vi "stdgetdbdataresults1.vi"(6 "connection reference":T1, 7 "type":string="s", 8 "ss ratio":u16(ring) items=["other", "36Cl"], 9 "wheelname":string, 10 "runletter":string, 11 "charge state":i32=2) -> (3 "seq std":dbl[][](array[numeric]), 4 "connection reference out":T1)   [LabVIEW 2016]
uses:
  <vilib>/addons/database/Connection.llb/Conn ObjectReference.ctl
  <vilib>/Analysis/baseanly.llb/Mean (DBL).vi
  <vilib>/addons/database/Connection.llb/Conn Execute.vi
  <vilib>/addons/database/Recordset.llb/Rec Fetch Recordset Data (R).vi
  <vilib>/addons/database/Recordset.llb/Rec Destroy - Connection.vi
  <vilib>/addons/database/NI_Database_API.lvlib
  <vilib>/Analysis/NI_AALBase.lvlib
panel:
  out "concatenated string":string
  out "seq result 2":dbl
  out "sorted array":dbl[](array[numeric])
  out "Array":dbl[][](array[numeric])
  out "position std result":string[][](array[string])
  out "std data":dbl[][][](array[numeric])
  out "seq result":dbl
  in  "SQL query 2":string
  out "error out 2":errorcluster
  out "sample data":string[][](array[string])
  out "recordset data":variant[][](array[variant])
  out "error out":errorcluster
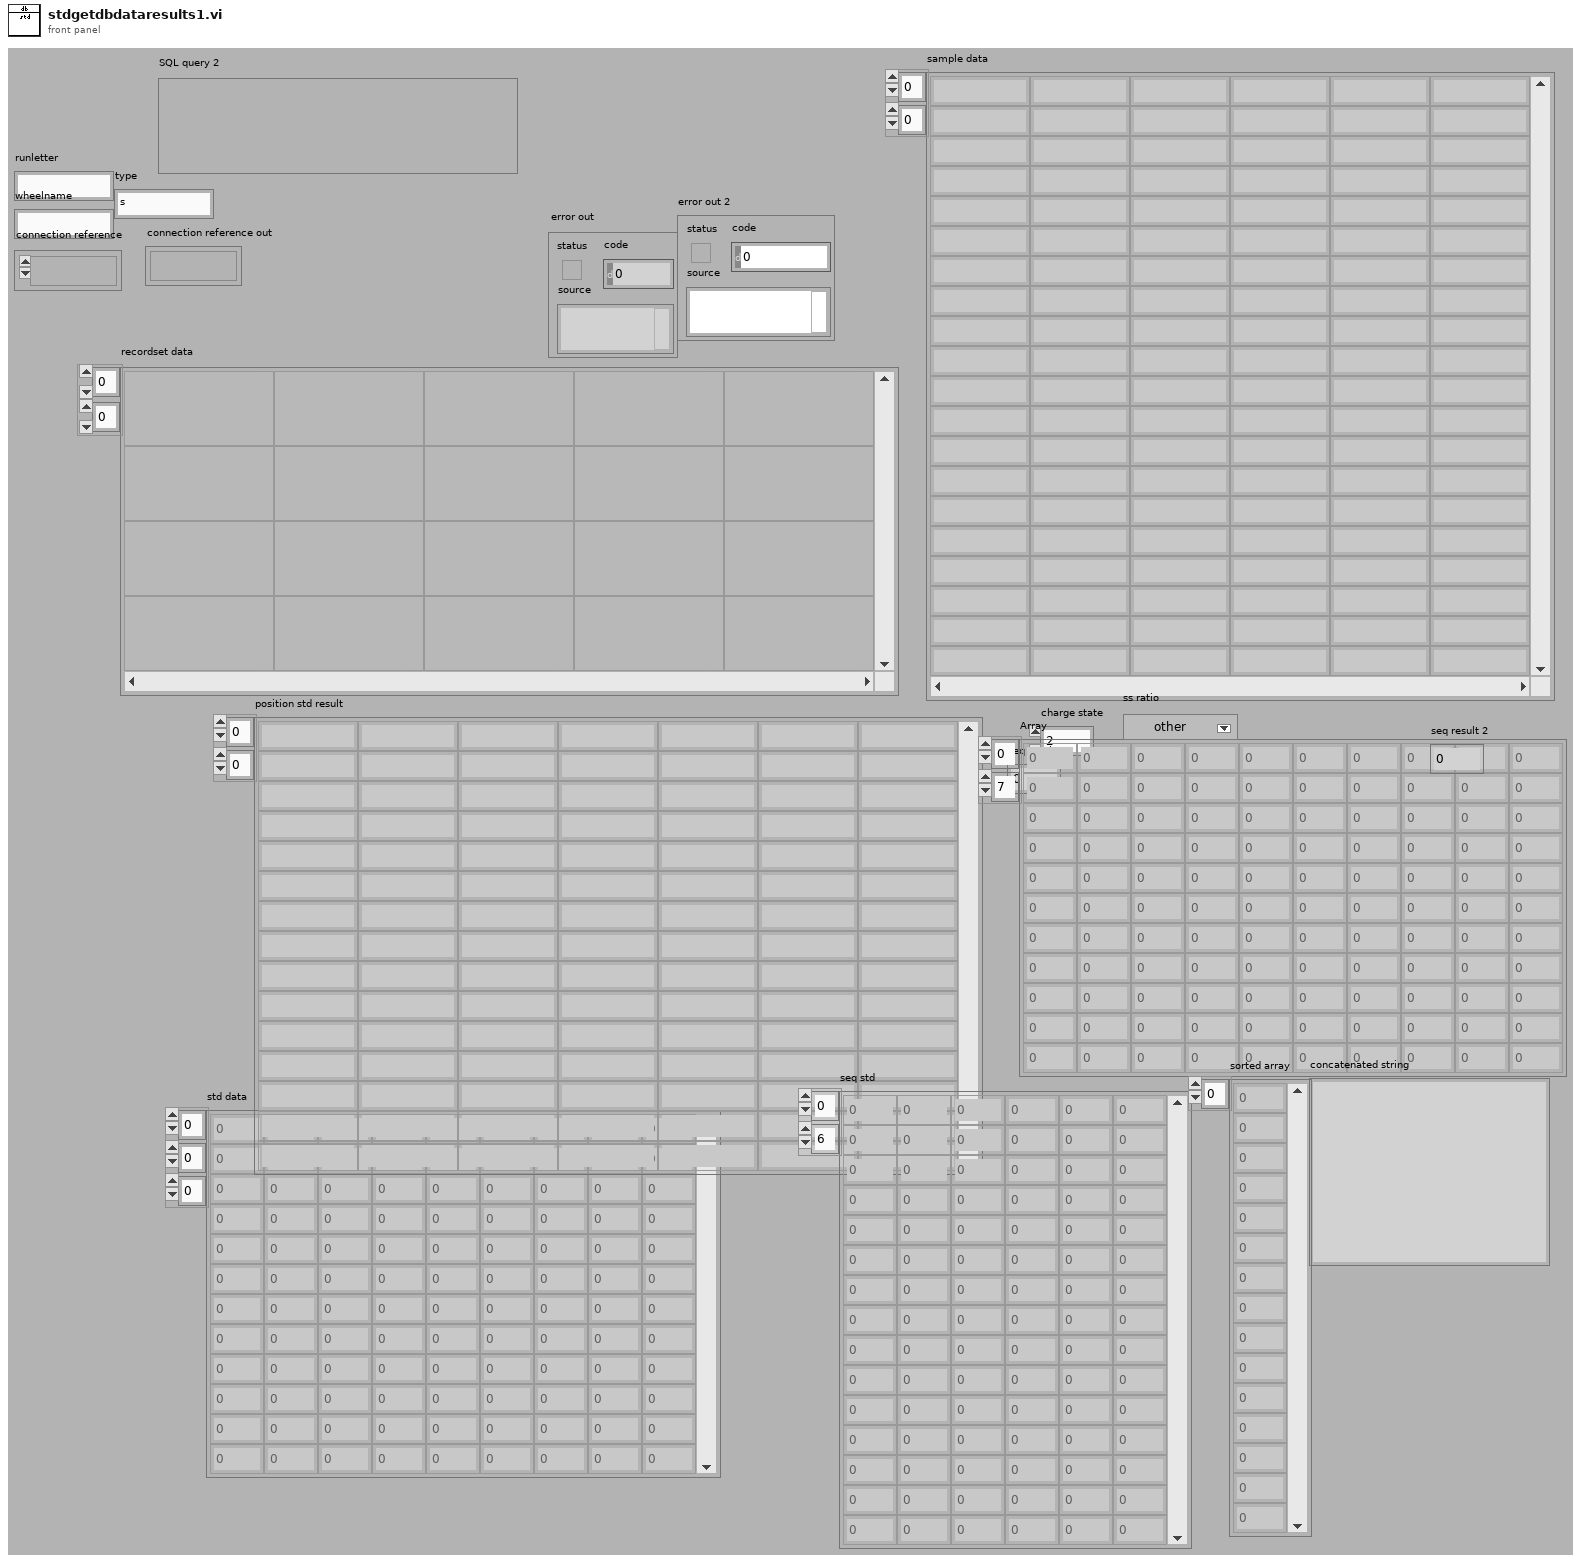
[diagram p1: front panel]
types:
  T1 = typedef "NI_Database_API.lvlib/Conn ObjectReference.ctl" = refnum<k1>
  T2 = typedef "NI_Database_API.lvlib/Rec ObjectReference.ctl" = refnum<k1>
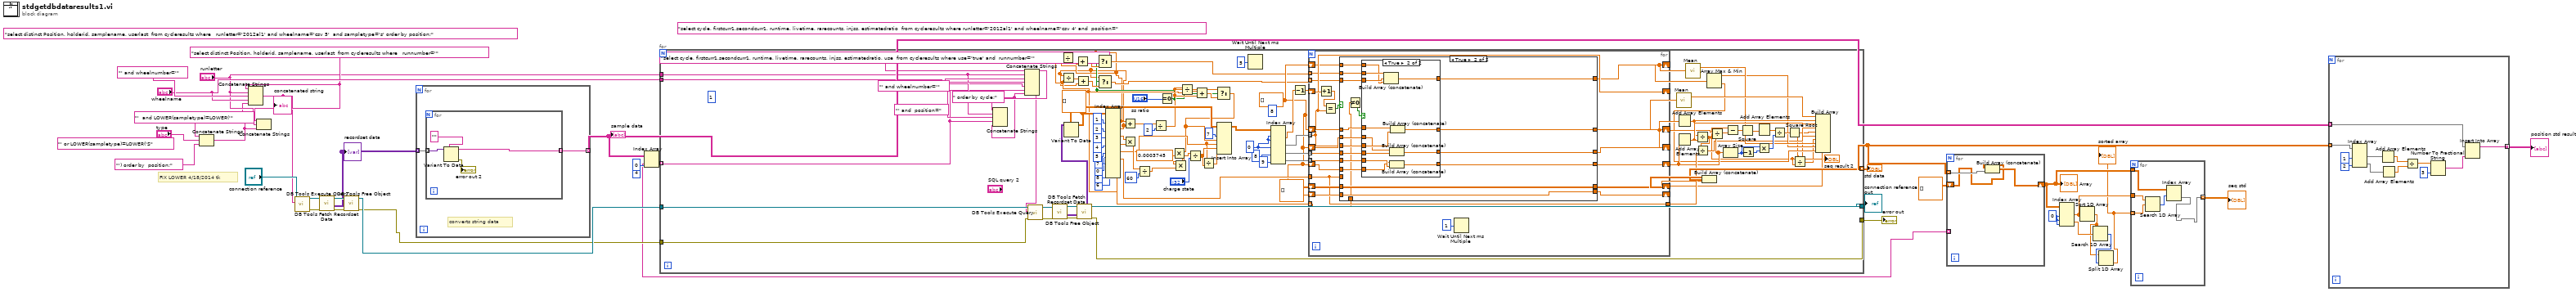
[diagram p0: block diagram]
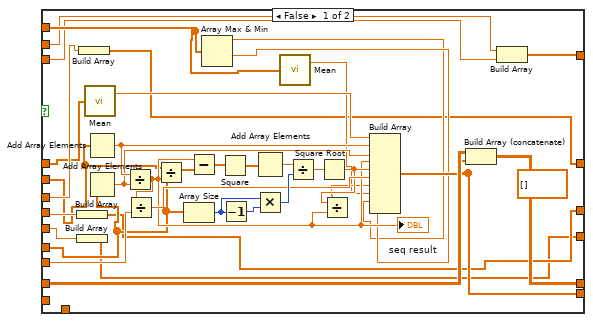
[diagram p2: hidden frame]
diagram:
  (unwired) "' or LOWER(sampletype)=LOWER('S" ("string")
  (unwired) "select cycle, firstcurr1,secondcurr1, runtime, livetime, rarecounts, injss, estimatedratio  from cycleresults where runletter='2012al1' and wheelname='csv 4' and  position=" ("SQL query 3")
  (unwired) "select distinct Position, holderid, samplename, userlast  from cycleresults where   runletter='2012al1' and wheelname='csv 5'  and sampletype='s' order by position;" ("SQL query get data name")
  w9 = "select distinct Position, holderid, samplename, userlast  from cycleresults where   runnumber='" ("SQL query get data name")
  w18 = 0 ("disabled index (col)")
  (unwired) 4 ("index (col)")
  (unwired) 1
  # "FIX LOWER 4/18/2014 tk"
  n1 = Concatenate Strings("'  and LOWER(sampletype)=LOWER('" ("SQL query get data name"), "type", "') order by  position;" ("SQL query get data name")) -> (w4:string)
  n2 = Concatenate Strings(w9, "runletter", "' and wheelnumber='" ("SQL query get data name"), "wheelname", w4) -> (w7:string)
  "concatenated string" <- w7
  n3 = Concatenate Strings(w9, "runletter", w4) -> ()  [unwired: 1 out]
  n4 = call-poly <vilib>:"DB Tools Execute Query.vi"("SQL query"=w7, "connection reference"="connection reference") -> ("error out"=w33:errorcluster, "recordset reference"=w32:T2)  [unwired: 6 in]
  n5 = call-poly <vilib>:"DB Tools Fetch Recordset Data.vi"("error in (no error)"=w33, "recordset reference"=w32) -> ("error out"=w31:errorcluster, "recordset data"=w29:variant[][], "recordset reference out"=w30:T2)  [unwired: 3 in]
  "recordset data" <- w29
  n6 = call-poly <vilib>:"DB Tools Free Object.vi"("error in (no error)"=w31, "recordset reference"=w30) -> ("error out"=w26:errorcluster, "connection reference"=w27:T1)  [unwired: 8 in]
  n7 = for {
    tunnel: w29 -> [w35] mode=indexing
    tunnel: [w34] -> w25 mode=indexing
    # "converts string data"
    n8 = for {
      tunnel: w35 -> [w39] mode=indexing
      tunnel: [w37] -> w34 mode=indexing
      n9 = Variant To Data(type="", Variant=w39) -> (data=w37:string, error out=→"error out 2":errorcluster)  [unwired: 1 in]
    }
  }
  "sample data" <- w25
  n10 = Index Array(array=w25, index (col)=0 ("disabled index (col)")) -> (element=w1:string[])  [unwired: 1 in]
  n11 = for {
    tunnel: w1 -> [w56] mode=indexing
    tunnel: w26 -> [w135]
    tunnel: w27 -> [w134]
    tunnel: [w131] -> w2
    tunnel: [w130] -> w10
    tunnel: [w100] -> w23 mode=indexing
    tunnel: "runletter" -> [w71]
    tunnel: "wheelname" -> [w73]
    w70 = "' and  position=" ("SQL query 3")
    w69 = " order by cycle;" ("string")
    w72 = "select cycle, firstcurr1,secondcurr1, runtime, livetime, rarecounts, injss, estimatedratio, use  from cycleresults where use='true' and  runnumber='" ("SQL query 3")
    w75 = dbl[] []
    w105 = 0 ("disabled index (col)")
    (unwired) 8 ("disabled index (col)")
    n12 = Concatenate Strings(w72, w71, w70, w56, w69) -> ()  [unwired: 1 out]
    n13 = Concatenate Strings(w72, w71, "' and wheelnumber='" ("SQL query 3"), w73, w70, w56, w69) -> (w68:string)
    n14 = call-poly <vilib>:"DB Tools Execute Query.vi"("error in (no error)"=w135, "SQL query"=w68, "connection reference"=w134) -> ("error out"=w133:errorcluster, "recordset reference"=w137:T2)  [unwired: 5 in]
    n15 = call-poly <vilib>:"DB Tools Fetch Recordset Data.vi"("error in (no error)"=w133, "recordset reference"=w137) -> ("error out"=w132:errorcluster, "recordset data"=w129:variant[][], "recordset reference out"=w136:T2)  [unwired: 3 in]
    n16 = Variant To Data(type=dbl[][] [], Variant=w129) -> (data=w113:dbl[][])  [unwired: 1 in, 1 out]
    n17 = call-poly <vilib>:"DB Tools Free Object.vi"("error in (no error)"=w132, "recordset reference"=w136) -> ("error out"=w131:errorcluster, "connection reference"=w130:T1)  [unwired: 8 in]
    n18 = Index Array(array=w113, index (col) #1=1 ("index (row)"), index (col) #2=2 ("disabled index (col)"), index (col) #3=3 ("index (col)"), index (col) #4=4 ("index (col)"), index (col) #5=5 ("index (col)"), index (row) #6=0 ("disabled index (row)"), index (col) #6=7 ("index (col)"), index (col) #7=8 ("index (col)"), index (col) #8=6 ("index (col)")) -> (element #1=w41:dbl[], element #2=w40:dbl[], element #3=w118:dbl[], element #4=w119:dbl[], element #5=w95:dbl[], element #6=w96:dbl, element #7=w58:dbl[], element #8=w45:dbl[])  [unwired: 7 in]
    n19 = Divide(x=w41, y=w45) -> (x/y=w49:dbl[])
    n20 = Divide(x=w40, y=w45) -> (x/y=w46:dbl[])
    n21 = Add(x=w49, y=w41) -> (x+y=w48:dbl[])
    n22 = Add(x=w46, y=w40) -> (x+y=w47:dbl[])
    n23 = Add(x=w41, y=w40) -> (x+y=w125:dbl[])
    n24 = Multiply(x=w118, y=w119) -> (x*y=w112:dbl[])
    n25 = Divide(x=w112, y=60) -> (x/y=w93:dbl[])
    n26 = Divide(x=w125, y=2) -> (x/y=w51:dbl[])
    n27 = Equal To 0?(x="ss ratio") -> (x = 0?=w43:bool)
    n28 = Select(t=w41, s=w43, f=w48) -> (s? t:f=w44:dbl[])
    n29 = Select(t=w40, s=w43, f=w47) -> (s? t:f=w42:dbl[])
    n30 = Divide(x=w51, y=w45) -> (x/y=w53:dbl[])
    n31 = Add(x=w53, y=w51) -> (x+y=w54:dbl[])
    n32 = Select(t=w51, s=w43, f=w54) -> (s? t:f=w50:dbl[])
    n33 = Multiply(x=w50, y=0.0003745) -> (x*y=w94:dbl[])
    n34 = Multiply(x=w94, y=w93) -> (x*y=w92:dbl[])
    n35 = Divide(x=w92, y="charge state") -> (x/y=w115:dbl[])
    n36 = Divide(x=w95, y=w115) -> (x/y=w114:dbl[])
    n37 = Insert Into Array(array=w113, index (col)=7 ("disabled index (col)"), new element #1=w50, new element #2=w95, new element #3=w115, new element #4=w114) -> (w111:dbl[][])  [unwired: 1 in]
    n38 = Wait Until Next ms Multiple(millisecond multiple=u32 5) -> ()  [unwired: 1 out]
    n39 = Index Array(array=w111, index (row) #1=w105, index (col) #1=w105, index (col) #2=w105, index (col) #3=8 ("index (col)"), index (col) #4=9 ("index (col)")) -> (element #1=w104:dbl, element #2=w106:dbl[], element #3=w108:dbl[], element #4=w107:dbl[])  [unwired: 3 in]
    n40 = Decrement(x=w104) -> (x-1=w103:dbl)
    n41 = for {
      tunnel: w106 -> [w147] mode=indexing
      tunnel: w108 -> [w157] mode=indexing
      tunnel: w107 -> [w156] mode=indexing
      shift-right: [w147] -> _
      shift-left: w103 -> [w160]
      shift-right: [w155] -> w80
      shift-left: w75 -> [w154]
      shift-right: [w152] -> w79
      shift-left: w75 -> [w151]
      shift-right: [w153] -> w77
      shift-left: w75 -> [w150]
      shift-right: [w149] -> w101
      shift-left: dbl[][] [] -> [w148]
      shift-right: [w146] -> _
      shift-left: w75 -> [w145]
      tunnel: w96 -> [w144]
      tunnel: [w144] -> w78
      tunnel: w44 -> [w142] mode=indexing
      tunnel: w42 -> [w143] mode=indexing
      shift-right: [w141] -> w66
      shift-left: w75 -> [w140]
      tunnel: w58 -> [w139] mode=indexing
      n42 = Increment(x=w160) -> (x+1=w159:dbl)
      n43 = Equal?(x=w159, y=w147) -> (x = y?=w158:bool)
      n44 = case shown="True" w158 {
        tunnel: w147 -> [w167 w212]
        tunnel: w157 -> [w179 w207]
        tunnel: w156 -> [w178 w208]
        tunnel: [w165 w211] -> w155
        tunnel: w154 -> [w166 w210]
        tunnel: [w161 w209] -> w153
        tunnel: [w162 w206] -> w152
        tunnel: w151 -> [w164 w205]
        tunnel: w150 -> [w163 w204]
        tunnel: [w192 w203] -> w149
        tunnel: w148 -> [w191 w203]
        tunnel: [w182 w202] -> w146
        tunnel: w145 -> [_ w202]
        tunnel: w144 -> [w181 _]
        tunnel: w143 -> [w169 w201]
        tunnel: w142 -> [w170 w200]
        tunnel: [w168 w199] -> w141
        tunnel: w140 -> [w174 w198]
        tunnel: w139 -> [_ w197]
        frame False {
          (unwired) dbl[] []
          n45 = Build Array(w179) -> (w162:dbl[])
          n46 = Build Array(w178) -> (w161:dbl[])
          n47 = Build Array(w167) -> (w165:dbl[])
          n48 = call-poly <vilib>:"Mean.vi"("X"=w166) -> ("mean"=w195:dbl)  [unwired: 1 out]
          n49 = Add Array Elements(numeric array=w164) -> (sum=w194:dbl)
          n50 = Add Array Elements(numeric array=w163) -> (sum=w193:dbl)
          n51 = Divide(x=w194, y=w193) -> (x/y=w176:dbl)
          "seq result" <- w176
          n52 = Divide(x=w176, y=w181) -> (x/y=w180:dbl)
          n53 = Divide(x=w164, y=w163) -> (x/y=w190:dbl[])
          n54 = Array Size(array=w163) -> (size(s)=w186:i32)
          n55 = Subtract(x=w176, y=w190) -> (x-y=w189:dbl[])
          n56 = Array Max & Min(array=w174) -> (max value=w171:dbl, min value=w172:dbl)  [unwired: 2 out]
          n57 = Square(x=w189) -> (x^2=w188:dbl[])
          n58 = Decrement(x=w186) -> (x-1=w187:i32)
          n59 = Add Array Elements(numeric array=w188) -> (sum=w184:dbl)
          n60 = Multiply(x=w186, y=w187) -> (x*y=w185:i32)
          n61 = call-poly <vilib>:"Mean.vi"("X"=w174) -> ("mean"=w173:dbl)  [unwired: 1 out]
          n62 = Divide(x=w184, y=w185) -> (x/y=w183:dbl)
          n63 = Square Root(x=w183) -> (sqrt(x)=w177:dbl)
          n64 = Divide(x=w177, y=w176) -> (x/y=w175:dbl)
          n65 = Build Array(w195, w194, w193, w176, w177, w180, w175, w173, w171, w172) -> (w182:dbl[])
          n66 = Build Array (concatenate)(w191, w182) -> (w192:dbl[][])
          n67 = Build Array(w170, w169) -> (w168:dbl[])
        }
        frame True {
          n68 = Not Equal To 0?(x=w197) -> (x != 0?=w196:bool)
          n69 = case shown="True" w196 {
            tunnel: w212 -> [_ w229]
            tunnel: [w215 w228] -> w211
            tunnel: w210 -> [w215 w227]
            tunnel: [w213 w226] -> w209
            tunnel: w208 -> [_ w225]
            tunnel: w207 -> [_ w224]
            tunnel: [w214 w223] -> w206
            tunnel: w205 -> [w214 w222]
            tunnel: w204 -> [w213 w221]
            tunnel: w201 -> [_ w220]
            tunnel: w200 -> [_ w219]
            tunnel: [w216 w218] -> w199
            tunnel: w198 -> [w216 w217]
            frame False {
            }
            frame True {
              n70 = Build Array (concatenate)(w219, w220, w217) -> (w218:dbl[])
              n71 = Build Array (concatenate)(w222, w224) -> (w223:dbl[])
              n72 = Build Array (concatenate)(w221, w225) -> (w226:dbl[])
              n73 = Build Array (concatenate)(w227, w229) -> (w228:dbl[])
            }
          }
        }
      }
      n74 = Wait Until Next ms Multiple(millisecond multiple=u32 1) -> ()  [unwired: 1 out]
    }
    n75 = call-poly <vilib>:"Mean.vi"("X"=w80) -> ("mean"=w81:dbl)  [unwired: 1 out]
    n76 = Add Array Elements(numeric array=w79) -> (sum=w82:dbl)
    n77 = Add Array Elements(numeric array=w77) -> (sum=w83:dbl)
    n78 = call-poly <vilib>:"Mean.vi"("X"=w66) -> ("mean"=w67:dbl)  [unwired: 1 out]
    n79 = Divide(x=w82, y=w83) -> (x/y=w62:dbl)
    "seq result 2" <- w62
    n80 = Divide(x=w62, y=w78) -> (x/y=w63:dbl)
    n81 = Array Max & Min(array=w66) -> (max value=w65:dbl, min value=w64:dbl)  [unwired: 2 out]
    n82 = Divide(x=w79, y=w77) -> (x/y=w84:dbl[])
    n83 = Array Size(array=w77) -> (size(s)=w88:i32)
    n84 = Subtract(x=w62, y=w84) -> (x-y=w85:dbl[])
    n85 = Square(x=w85) -> (x^2=w86:dbl[])
    n86 = Decrement(x=w88) -> (x-1=w87:i32)
    n87 = Add Array Elements(numeric array=w86) -> (sum=w90:dbl)
    n88 = Multiply(x=w88, y=w87) -> (x*y=w89:i32)
    n89 = Divide(x=w90, y=w89) -> (x/y=w91:dbl)
    n90 = Square Root(x=w91) -> (sqrt(x)=w61:dbl)
    n91 = Divide(x=w61, y=w62) -> (x/y=w60:dbl)
    n92 = Build Array(w81, w82, w83, w62, w61, w63, w60, w67, w65, w64) -> (w76:dbl[])
    n93 = Build Array (concatenate)(w101, w76) -> (w100:dbl[][])
  }
  "error out" <- w2
  "std data" <- w23
  "connection reference out" <- w10
  n94 = for {
    tunnel: w23 -> [w231] mode=indexing
    shift-right: [w232] -> w20
    shift-left: dbl[][] [] -> [w230]
    tunnel: w1 -> [_] mode=indexing
    n95 = Build Array (concatenate)(w230, w231) -> (w232:dbl[][])
  }
  "Array" <- w20
  n96 = Index Array(array=w20, index (col) #1=w18, index (row) #2=w18, index (col) #2=w18) -> (element #1=w21:dbl[], element #2=w17:dbl)  [unwired: 1 in]
  n97 = Sort 1D Array(array=w21) -> (sorted array=w15:dbl[])
  n98 = Search 1D Array(1D array=w15, element=w17) -> (index of element=w16:i32)  [unwired: 1 in]
  n99 = Split 1D Array(array=w15, index=w16) -> (second subarray=w14:dbl[])  [unwired: 1 out]
  "sorted array" <- w14
  n100 = for {
    tunnel: w14 -> [w236] mode=indexing
    tunnel: w21 -> [w237]
    tunnel: w20 -> [w235]
    tunnel: [w233] -> w19 mode=indexing
    n101 = Search 1D Array(1D array=w237, element=w236) -> (index of element=w234:i32)  [unwired: 1 in]
    n102 = Index Array(array=w235, index (row)=w234) -> (element=w233:dbl[])  [unwired: 1 in]
  }
  "seq std" <- w19
  n103 = for {
    tunnel: w23 -> [w249] mode=indexing
    tunnel: w25 -> [w240] mode=indexing
    tunnel: [w238] -> w24 mode=indexing
    n104 = Index Array(array=w249, index (col) #1=1 ("disabled index (col)"), index (col) #2=2 ("index (col)")) -> (element #1=w245:dbl[], element #2=w246:dbl[])  [unwired: 2 in]
    n105 = Add Array Elements(numeric array=w245) -> (sum=w243:dbl)
    n106 = Add Array Elements(numeric array=w246) -> (sum=w244:dbl)
    n107 = Divide(x=w243, y=w244) -> (x/y=w242:dbl)
    n108 = Number To Fractional String(number=w242, precision (6)=i16 3) -> (F-format string=w239:string)  [unwired: 2 in]
    n109 = Insert Into Array(array=w240, new element=w239) -> (w238:string[])  [unwired: 1 in]
  }
  "position std result" <- w24
